vi "Format Digital Pattern Plot.vi"(10 "Rotations":u16, 11 "Patterns":T1[](array[typedef])) -> (3 "Patterns":T1[](array[typedef]))   [LabVIEW 2020, in "Engine Simulation Toolkit System Explorer.lvlib"]
uses:
  Engine Simulation Toolkit System Explorer.lvlib
  Digital Pattern Expanded.ctl
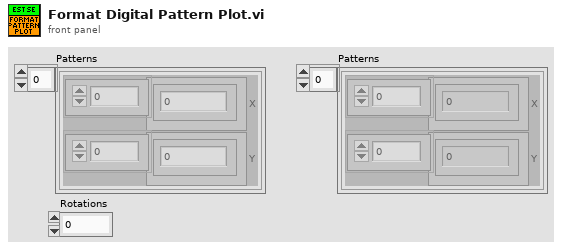
[diagram p1: front panel]
types:
  T1 = typedef "Engine Simulation Toolkit System Explorer.lvlib/Digital Pattern Expanded.ctl" = cluster{"X":dbl[], "Y":dbl[]}
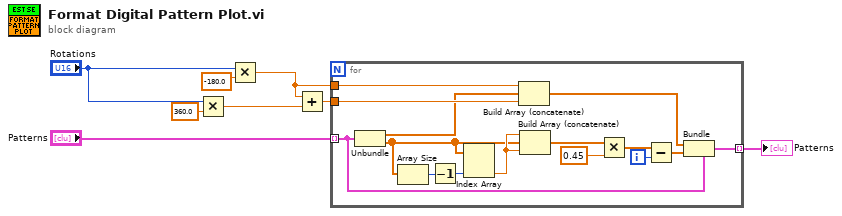
[diagram p0: block diagram]
diagram:
  n1 = Multiply(x="Rotations", y=360.0) -> (x*y=w4:dbl)
  n2 = Multiply(x="Rotations", y=-180.0) -> (x*y=w1:dbl)
  n3 = Add(x=w1, y=w4) -> (x+y=w5:dbl)
  n4 = for {
    tunnel: "Patterns" -> [w21] mode=indexing
    tunnel: [w19] -> w8 mode=indexing
    tunnel: w1 -> [w15]
    tunnel: w5 -> [w14]
    i -> [w20]
    n5 = Unbundle(w21) -> ("X"=w12:dbl[], "Y"=w11:dbl[])
    n6 = Array Size(array=w11) -> (size(s)=w17:i32)
    n7 = Decrement(x=w17) -> (x-1=w16:i32)
    n8 = Index Array(array=w11, index #2=w16) -> (element #2=w13:dbl)  [unwired: 1 in, 1 out]
    n9 = Build Array (concatenate)(w15, w12, w14) -> (w9:dbl[])
    n10 = Build Array (concatenate)(w13, w11, w13) -> (w18:dbl[])
    n11 = Multiply(x=w18, y=0.45) -> (x*y=w22:dbl[])
    n12 = Subtract(x=w22, y=w20) -> (x-y=w10:dbl[])
    n13 = Bundle(cluster=w21, "X"=w9, "Y"=w10) -> (w19:T1)
  }
  "Patterns" <- w8
